vi "WDT Append Waveforms SGL (Modified).vi"(8 "error in (no error)":errorcluster, 10 "waveform B":waveform(sgl), 11 "waveform A":waveform(sgl)) -> (0 "error out":errorcluster, 3 "waveform out":waveform(sgl))   [LabVIEW 2012, in "Data Acquisition.lvlib" / "DAQ Actor.lvclass"]
doc: "Appends <B>waveform B</B> to the end of <B>waveform A</B>. If the sampling rates do not match, the error cluster returns an error. The trigger time of <B>waveform B</B> is ignored. The data type of the Y component of <B>waveform A</B> and <B>waveform B</B> determines the polymorphic instance to use or you can manually select the instance."
uses:
  DAQ Actor.lvclass
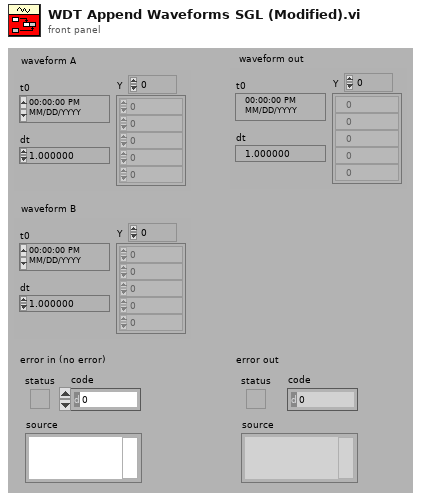
[diagram p1: front panel]
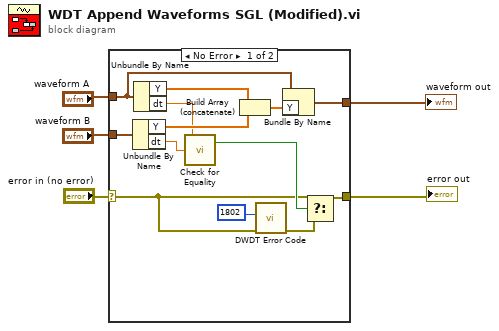
[diagram p0: block diagram]
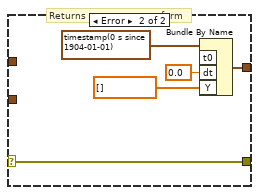
[diagram p2: hidden frame]
diagram:
  n1 = case shown="No Error" "error in (no error)" {
    selector: "error in (no error)" -> [w6 w23]
    tunnel: "waveform A" -> [w15 _]
    tunnel: "waveform B" -> [w18 _]
    tunnel: [w14 w22] -> w5
    tunnel: [w10 w23] -> w1
    frame No Error {
      n2 = Unbundle By Name(w18) -> ("Y"=w16:sgl[], "dt"=w12:dbl)
      n3 = Unbundle By Name(w15) -> ("Y"=w17:sgl[], "dt"=w13:dbl)
      n4 = call <vilib>:"Check for Equality.vi"("n2"=w12, "n1"=w13) -> ("equal?"=w9:bool)  [unwired: 2 out]
      n5 = Build Array (concatenate)(w17, w16) -> (w11:sgl[])
      n6 = call <vilib>:"DWDT Error Code.vi"("error in (no error)"=w6, "error code"=1802) -> ("error out"=w7:errorcluster)  [unwired: 9 out]
      n7 = Bundle By Name(cluster=w15, "Y"=w11) -> (w14:waveform(sgl))
      n8 = Select(t=w6, s=w9, f=w7) -> (s? t:f=w10:errorcluster)
    }
    frame Error {
      # "Returns an empty waveform"
      # "Incoming Error"
      n9 = Bundle By Name("t0"=timestamp(0 s since 1904-01-01), "dt"=0.0, "Y"=dbl[] []) -> (w22:waveform(dbl))  [unwired: 1 out]
    }
  }
  "waveform out" <- w5
  "error out" <- w1
